vi "Clear.vi"(8 "error in (no error)":errorcluster, 11 "Logger Level in":refnum<class "Logger Level.lvclass">) -> (0 "error out":errorcluster, 3 "Logger Level out":refnum<class "Logger Level.lvclass">)   [LabVIEW 2020, in "Logger Level.lvlib" / "Logger Level.lvclass"]
uses:
  Logger Level.lvclass
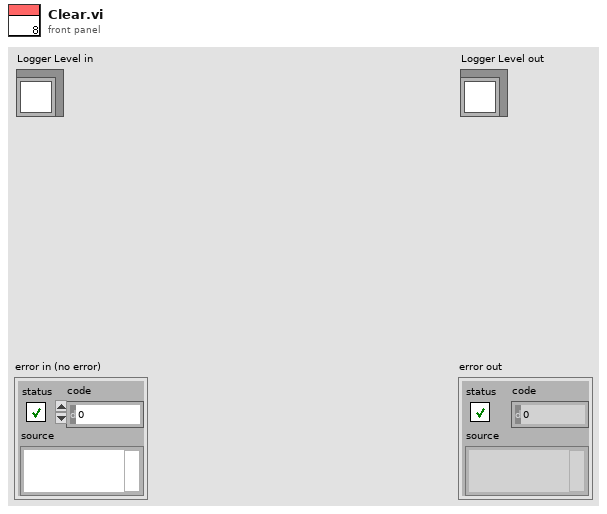
[diagram p1: front panel]
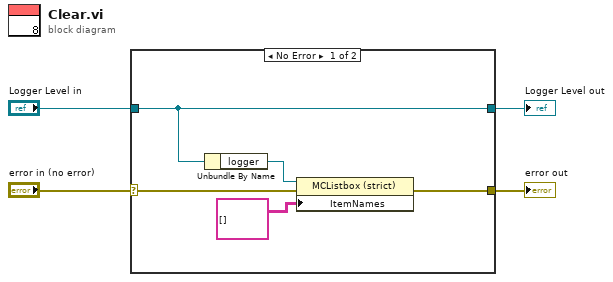
[diagram p0: block diagram]
diagram:
  n1 = case shown="No Error" "error in (no error)" {
    selector: "error in (no error)" -> [w8 w11]
    tunnel: [w5 w11] -> w3
    tunnel: [w9 w10] -> w1
    tunnel: "Logger Level in" -> [w9 w10]
    frame No Error {
      n2 = Unbundle By Name(w9) -> ("logger"=w7:refnum<vi>)
      n3 = property class="MCListbox (strict)"(reference=w7, error in=w8, "ItemNames"=string[][] [] ("Item Names")) -> (error out=w5:errorcluster)  [unwired: 1 out]
    }
    frame Error {
    }
  }
  "error out" <- w3
  "Logger Level out" <- w1
